vi "kalman filter demo.vi"() -> ()   [LabVIEW 2012]
uses:
  <vilib>/ptbypt/NI_PtbyPt.lvlib
panel:
  out "millisecond timer value":u32
  out "Waveform Chart":cluster{"dx/dt":dbl, "x_out":dbl}(graph)
  in  "r":dbl=50.0
  in  "q":dbl=0.1
  in  "stop":bool
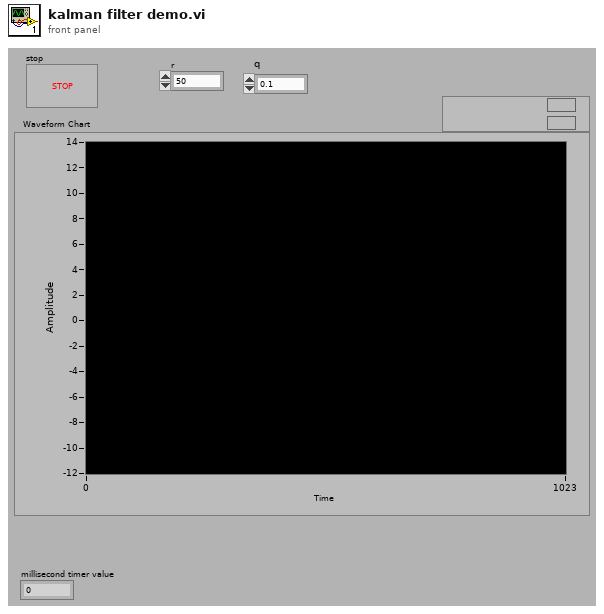
[diagram p1: front panel]
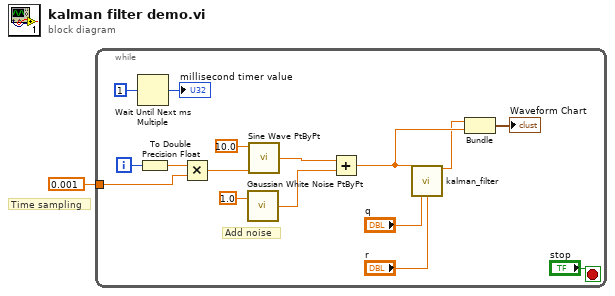
[diagram p0: block diagram]
diagram:
  # "Time sampling"
  n1 = while {
    tunnel: 0.001 -> [w5]
    i -> [w14]
    stop <- "stop" stop-if-true
    # "Add noise"
    n2 = Wait Until Next ms Multiple(millisecond multiple=u32 1) -> (millisecond timer value=→"millisecond timer value":u32)
    n3 = To Double Precision Float(number=w14) -> (double precision float=w6:dbl)
    n4 = Multiply(x=w6, y=w5) -> (x*y=w13:dbl)
    n5 = call <vilib>:"Gaussian White Noise PtByPt.vi"("standard deviation"=1.0) -> ("Gaussian white noise"=w7:dbl)  [unwired: 2 in]
    n6 = call <vilib>:"Sine Wave PtByPt.vi"("time"=w13, "amplitude"=10.0) -> ("sine wave"=w8:dbl)  [unwired: 2 in]
    n7 = Add(x=w8, y=w7) -> (x+y=w3:dbl)
    n8 = call "kalman_filter.vi"("measured value"=w3, "q"="q", "r"="r") -> ("x_out"=w2:dbl)  [unwired: 10 in, 2 out]
    n9 = Bundle("x_out"=w2, w3) -> (→"Waveform Chart":cluster{"x_out":dbl, dbl})  [unwired: 1 in]
  }
